vi "Untitled 1.vi"() -> ()   [LabVIEW 2020]
uses:
  Libraries/Graph Module/Graph Module.lvlib
  <vilib>/vision/NI_Vision_Development_Module.lvlib
panel:
  out "Image Display":T1(plugin-control)
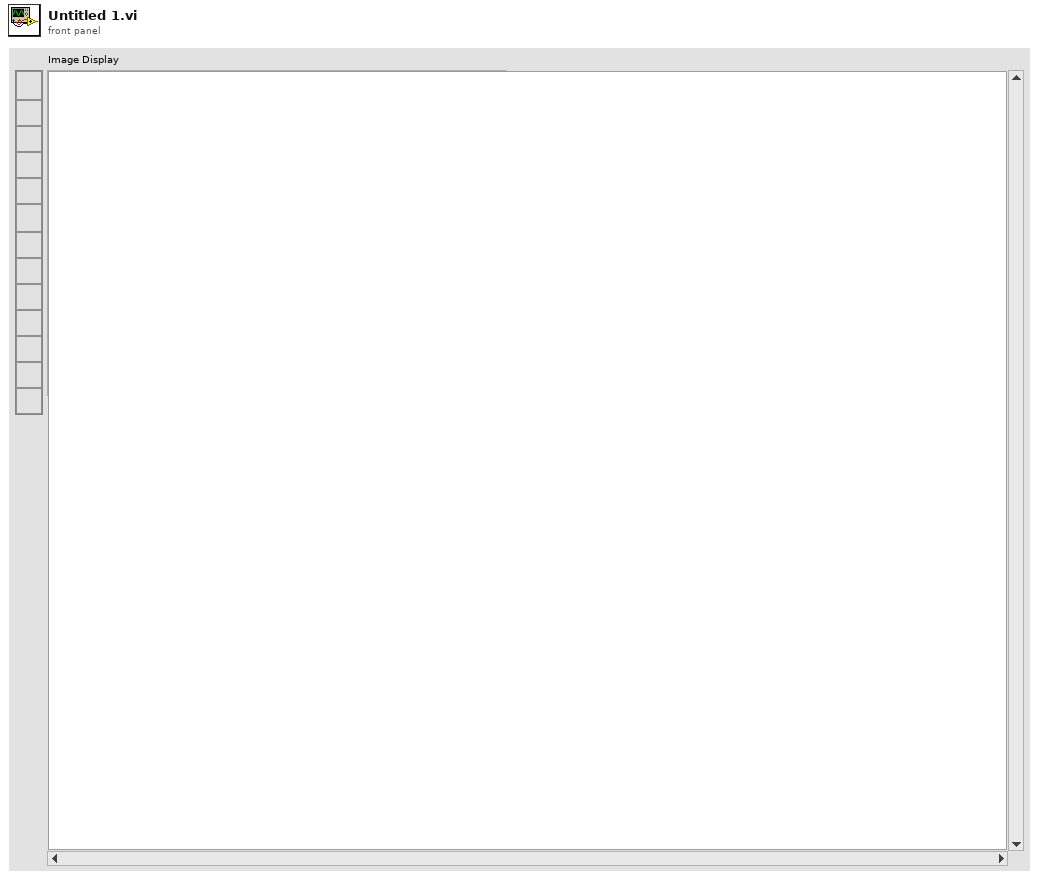
[diagram p1: front panel]
types:
  T1 = typedef "IMAQ Image.ctl" = refnum<image>
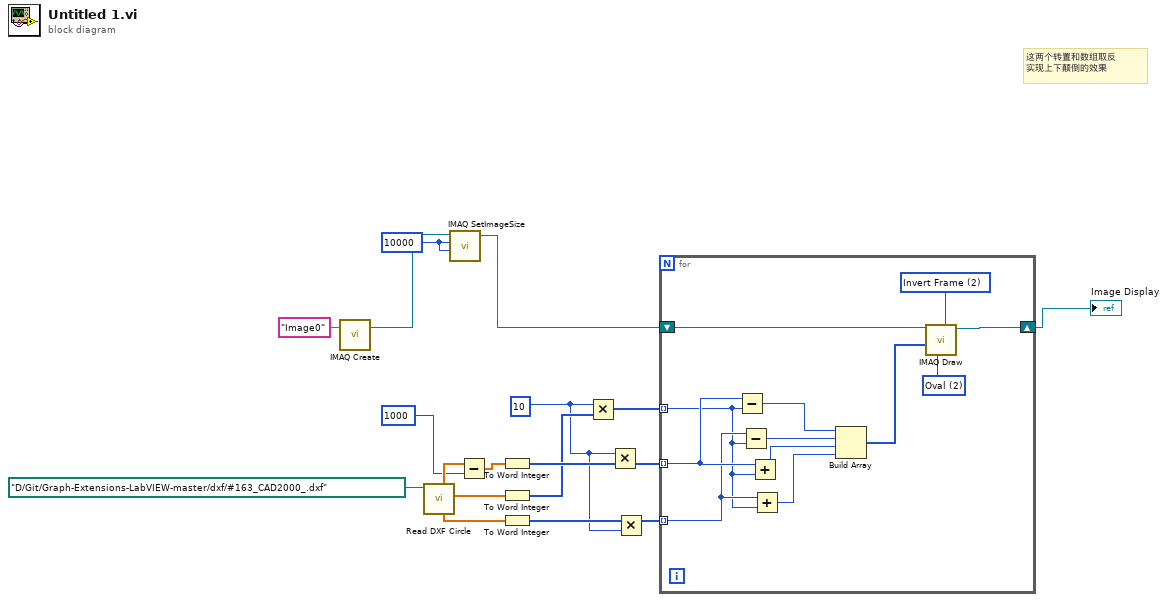
[diagram p0: block diagram]
diagram:
  w7 = 10000 ("X Resolution")
  w4 = 10
  # "这两个转置和数组取反\n实现上下颠倒的效果"
  n1 = call "IMAQ Create"("Image Name"="Image0") -> ("New Image"=w9:T1)  [unwired: 4 in, 1 out]
  n2 = call "Read DXF Circle.vi"("path"=path "D:/Git/Graph-Extensions-LabVIEW-master/dxf/#163_CAD2000_.dxf") -> ("Radius"=w1:dbl[], "Y"=w17:dbl[], "X"=w18:dbl[])  [unwired: 6 in, 2 out]
  n3 = call "IMAQ SetImageSize"("Y Resolution"=w7, "X Resolution"=w7, "Image"=w9) -> ("Image Out"=w8:T1)  [unwired: 2 in, 1 out]
  n4 = Subtract(x=w18, y=1000) -> (x-y=w3:dbl[])
  n5 = To Word Integer(number=w3) -> (16bit integer=w15:i16[])
  n6 = To Word Integer(number=w1) -> (16bit integer=w14:i16[])
  n7 = To Word Integer(number=w17) -> (16bit integer=w13:i16[])
  n8 = Multiply(x=w4, y=w14) -> (x*y=w11:i32[])
  n9 = Multiply(x=w4, y=w15) -> (x*y=w6:i32[])
  n10 = Multiply(x=w13, y=w4) -> (x*y=w5:i32[])
  n11 = for {
    tunnel: w11 -> [w25] mode=indexing
    tunnel: w6 -> [w27] mode=indexing
    tunnel: w5 -> [w26] mode=indexing
    shift-right: [w21] -> w10
    shift-left: w8 -> [w20]
    w19 = u16 2 items=["Frame", "Paint", "Invert Frame", "Invert Paint"] ("Draw Mode")
    w30 = u16 2 items=["Line", "Rectangle", "Oval"] ("Shape to draw")
    n12 = Subtract(x=w27, y=w25) -> (x-y=w29:i32)
    n13 = Subtract(x=w26, y=w25) -> (x-y=w28:i32)
    n14 = Add(x=w27, y=w25) -> (x+y=w24:i32)
    n15 = Add(x=w26, y=w25) -> (x+y=w23:i32)
    n16 = Build Array(w29, w28, w24, w23) -> (w22:i32[])
    n17 = call "IMAQ Draw"("Draw Mode"=w19, "Shape to draw"=w30, "Coordinates"=w22, "Image Src"=w20) -> ("Image Dst Out"=w21:T1)  [unwired: 6 in, 1 out]
  }
  "Image Display" <- w10
